vi "(Challenge) Read Delimited File into VI.vi"() -> ()   [LabVIEW 2019]
uses:
  <vilib>/Utility/file.llb/Read Delimited Spreadsheet (string).vi
  <vilib>/Utility/file.llb/Read Delimited Spreadsheet (DBL).vi
panel:
  out "Max Values Per Channel":dbl[](array[numeric])
  out "Min Values Per Channel":dbl[](array[numeric])
  out "Waveform Graph":dbl[][](graph)
  out "Data with first line header deleted":dbl[][](array[numeric])
  out "First row (header strings)":string[](array[string])
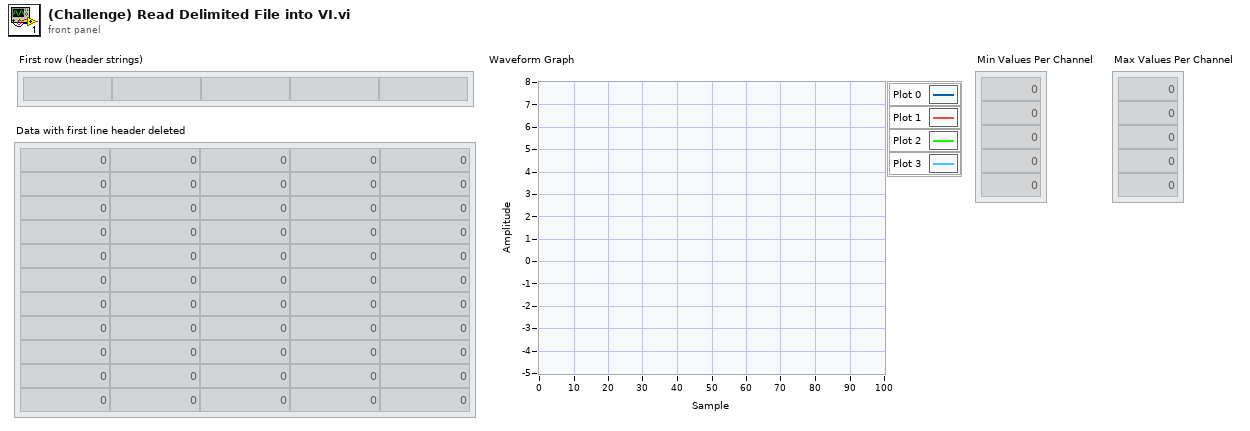
[diagram p1: front panel]
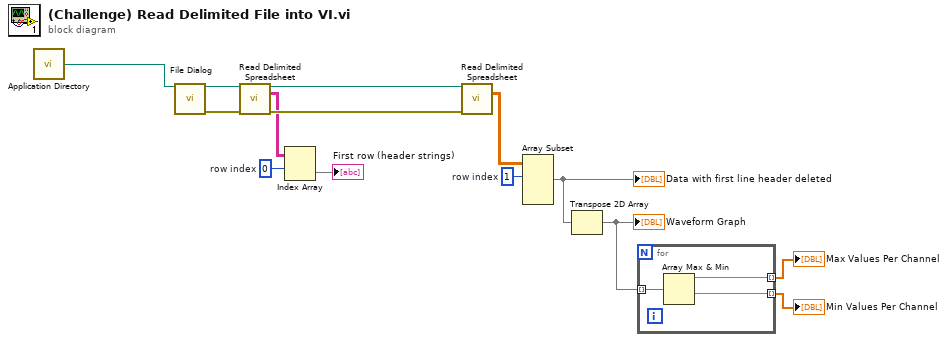
[diagram p0: block diagram]
diagram:
  w6 = 1  # row index
  w8 = 0  # row index
  n1 = call <vilib>:"Application Directory.vi"() -> ("Application Directory"=w14:path)
  n2 = call "File Dialog"("start path"=w14) -> ("selected path"=w13:path, "error out"=w12:errorcluster)  [unwired: 11 in, 2 out]
  n3 = call-poly <vilib>:"Read Delimited Spreadsheet.vi"("file path (dialog if empty)"=w13, "error in (no error)"=w12) -> ("new file path (Not A Path if cancelled)"=w11:path, "all rows"=w9:string[][], "error out"=w10:errorcluster)  [unwired: 8 in, 3 out]
  n4 = Index Array "Index Array"(array=w9, index (row)=w8) -> (element=→"First row (header strings)":string[])  [unwired: 1 in]
  n5 = call-poly <vilib>:"Read Delimited Spreadsheet.vi"("file path (dialog if empty)"=w11, "error in (no error)"=w10) -> ("all rows"=w7:dbl[][])  [unwired: 8 in, 5 out]
  n6 = Array Subset "Array Subset"(array=w7, index (row)=w6) -> (w4:dbl[][])  [unwired: 3 in]
  "Data with first line header deleted" <- w4
  n7 = Transpose 2D Array(2D array=w4) -> (transposed array=w3:dbl[][])
  "Waveform Graph" <- w3
  n8 = for {
    tunnel: w3 -> [w17] mode=indexing
    tunnel: [w16] -> w1 mode=indexing
    tunnel: [w15] -> w2 mode=indexing
    n9 = Array Max & Min(array=w17) -> (max value=w16:dbl, min value=w15:dbl)  [unwired: 2 out]
  }
  "Min Values Per Channel" <- w2
  "Max Values Per Channel" <- w1
